vi "Read Supported Instruments.vi"(8 "error in (no error)":errorcluster, 11 "Configuration in":refnum<class "Configuration.lvclass">) -> (0 "error out":errorcluster, 2 "Instruments":string[](array[string]), 3 "Configuration out":refnum<class "Configuration.lvclass">, 5 "Base Path":path=path "C:/Users/Public/Documents/Development/builds/Instruments")   [LabVIEW 2023, in "Configuration.lvlib" / "Configuration.lvclass"]
uses:
  Library/Configuration.lvclass
  Library/Configuration.lvclass/Configuration.ctl
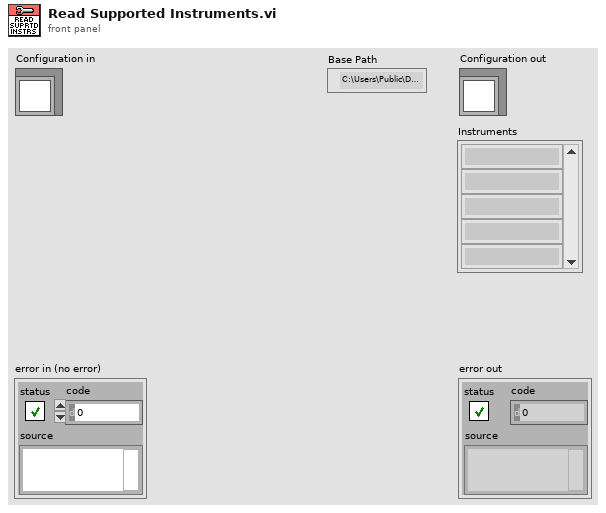
[diagram p1: front panel]
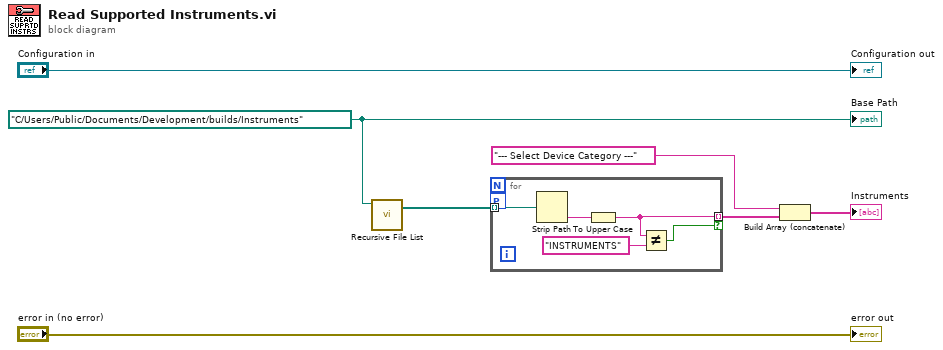
[diagram p0: block diagram]
diagram:
  w5 = path "C:/Users/Public/Documents/Development/builds/Instruments"
  n1 = call <vilib>:"Recursive File List.vi"("Folder Path"=w5) -> ("All Folders"=w4:path[])  [unwired: 6 in, 4 out]
  n2 = for {
    tunnel: w4 -> [w9] mode=indexing
    tunnel: [w11] -> w3 mode=indexing if=w8
    workers-P: _ -> [_]
    n3 = Strip Path(path=w9) -> (name=w12:string)  [unwired: 1 out]
    n4 = To Upper Case(1:w12) -> (0:w11:string)
    n5 = Not Equal?(x=w11, y="INSTRUMENTS") -> (x != y?=w8:bool)
  }
  n6 = Build Array (concatenate)("--- Select Device Category ---", w3) -> (→"Instruments":string[])
  "error out" <- "error in (no error)"
  "Configuration out" <- "Configuration in"
  "Base Path" <- w5
